vi "Launch Service Mode.vi"(8 "error in (no error)":errorcluster, 11 "Top Level in":refnum<class "Top Level.lvclass">) -> (0 "error out":errorcluster, 3 "Top Level out":refnum<class "Top Level.lvclass">)   [LabVIEW 2021, in "Top Level.lvlib" / "Top Level.lvclass"]
uses:
  Top Level.lvclass
  C:/Program Files/National Instruments/LabVIEW 2021/vi.lib/MGI/Panel Manager/Panel Actor/Panel Actor/Panel Actor.lvclass
  Service/Service.lvclass
  Top Level.lvclass/Top Level.ctl
  <vilib>/MGI/Panel Manager/Panel/Panel/Window/Window.lvclass
  C:/Program Files/National Instruments/LabVIEW 2021/vi.lib/MGI/Panel Manager/Panel/Panel/Panel.lvclass
  <vilib>/MGI/Panel Manager/Panel/Panel/Window/Window.vi
  <vilib>/MGI/Panel Manager/Panel Actor/Panel Actor/Panel Actor.lvclass
  <vilib>/MGI/Panel Manager/Panel/Panel.lvlib
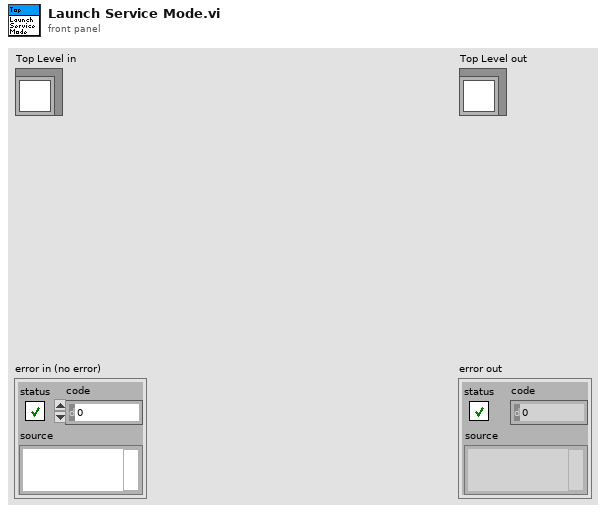
[diagram p1: front panel]
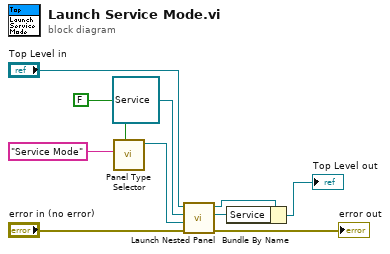
[diagram p0: block diagram]
diagram:
  n1 = call-poly <vilib>:"Panel Type Selector.vi"("Autoshow? (T)"=FALSE, "Default Title"="Service Mode") -> ("Window out"=w9:refnum<class "Window.lvclass">)  [unwired: 8 in, 1 out]
  n2 = call <vilib>:"Launch Nested Panel.vi"("error in (no error)"="error in (no error)", "Panel"=w9, "Nested Panel Actor"=refnum<class "Service.lvclass"> refnum ("Service.lvlib:Service.lvclass"), "Panel Actor in"="Top Level in") -> ("error out"=→"error out":errorcluster, "Nested Actor's Enqueuer"=w7:refnum<class "Message Enqueuer.lvclass">, "Panel Actor out"=w10:refnum<class "Top Level.lvclass">)  [unwired: 4 in, 1 out]
  n3 = Bundle By Name(cluster=w10, "Service"=w7) -> (→"Top Level out":refnum<class "Top Level.lvclass">)
